vi "Climber_Hardware_Globals.vi"() -> ()   [LabVIEW 2020]
panel:
  in  "Elevator_Right":string="Elevator_Right"
  in  "Elevator_Left":string="Elevator_Left"
  in  "Outer_Arm_Pivot":string="Outer_Arm_Pivot"
  in  "Inner_Arm_Pivot":string="Inner_Arm_Pivot"
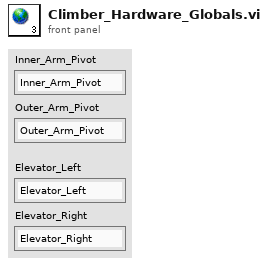
[diagram p1: front panel]
diagram:
